vi "Skip.vi"(7 "Description":string, 8 "error in (no error)":errorcluster, 9 "Message":string, 11 "LUnit Test Case In":refnum<class "LUnit Test Case.lvclass">) -> (0 "error out":errorcluster, 3 "LUnit Test Case Out":refnum<class "LUnit Test Case.lvclass">)   [LabVIEW 2020, in "LUnit Test Case.lvclass"]
doc: "Ignores results from the calling test method when evaluating the test case result. A description and message may be provided.\nThis method should be added after any assertion in a test to skip the result from these assertions."
uses:
  LUnit Test Case.lvclass
  Result/Type.ctl
  Result/Result.ctl
  Result/Status.ctl
  LUnit Test Case.lvclass/LUnit Test Case.ctl
  Result/Result.lvlib
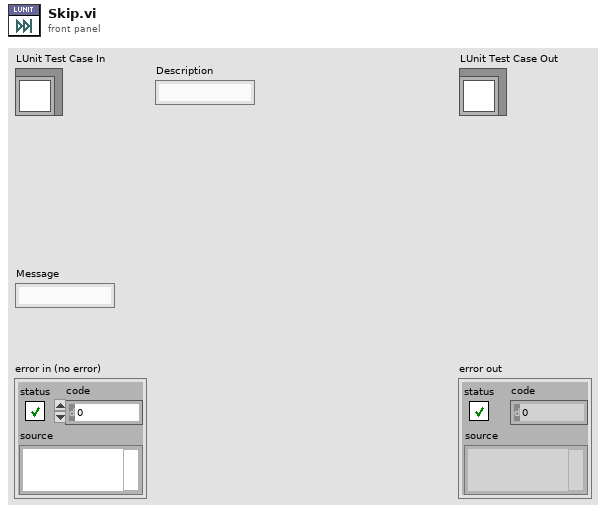
[diagram p1: front panel]
types:
  T1 = typedef "Result.lvlib/Type.ctl" = enum16{"Test Case", "Test Suite", "Test Run", "Pass", "Fail", "Skip", "Pass if", "Fail if", "Pass if Error", "Fail if Error", "Pass if Equal", "Fail if Equal"}
  T2 = typedef "Result.lvlib/Result.ctl" = cluster{"Name":string, "Description":string, "Status":T3, "Result Type":T1, "Execution Time":dbl, "Data":cluster{"Expected":variant, "Actual":variant, "Delta":variant}}
  T3 = typedef "Result.lvlib/Status.ctl" = enum16{"", "Passed", "Failed", "Error", "Skipped", "Setup Error", "Broken", "Teardown Error"}
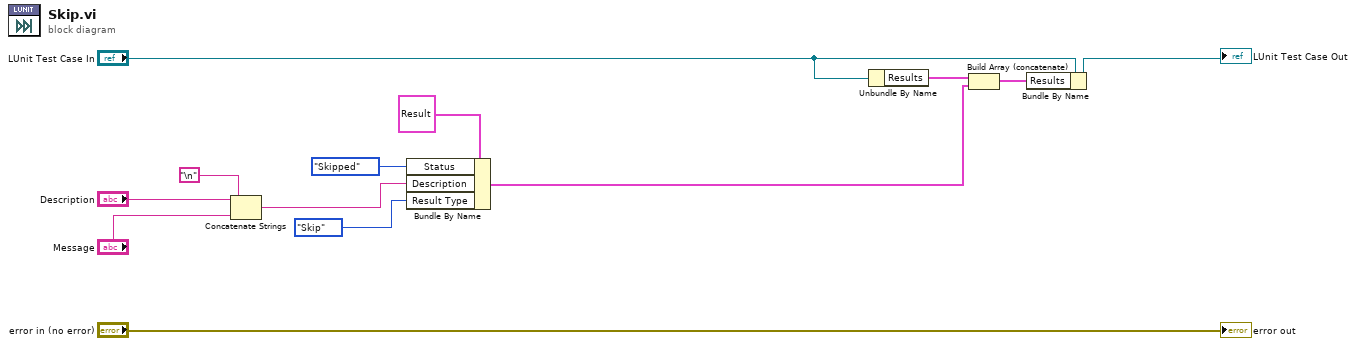
[diagram p0: block diagram]
diagram:
  n1 = Concatenate Strings("Description", "\n", "Message") -> (w3:string)
  n2 = Bundle By Name(cluster=T2 {"Name"="", "Description"="", "Status"=enum."Passed", "Result Type"=enum."Test Case", "Execution Time"=0.0, "Data"={"Expected"=variant, "Actual"=variant, "Delta"=variant}} ("Temporary Assertion Result"), "Status"=Status."Skipped", "Description"=w3, "Result Type"=Type."Skip") -> (w10:T2)
  n3 = Unbundle By Name("LUnit Test Case In") -> ("Results"=w6:T2[])
  n4 = Build Array (concatenate)(w6, w10) -> (w4:T2[])
  n5 = Bundle By Name(cluster="LUnit Test Case In", "Results"=w4) -> (→"LUnit Test Case Out":refnum<class "LUnit Test Case.lvclass">)
  "error out" <- "error in (no error)"
